vi "Image Aqq Module Test.vi"() -> ()   [LabVIEW 2015]
uses:
  <vilib>/vision/Image Controls.llb/IMAQ Image.ctl
panel:
  out "Image":T1(plugin-control)
  in  "Stop":bool
  in  "Pause":bool
  in  "Start":bool
  # "Image Stream"
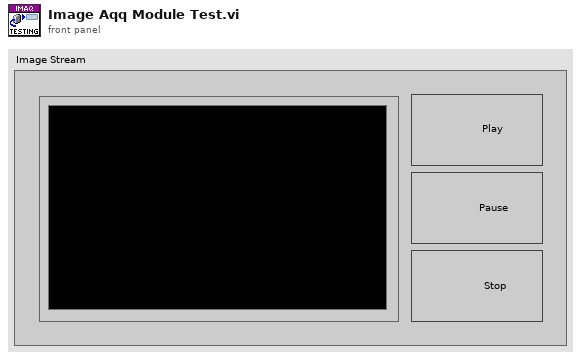
[diagram p1: front panel]
types:
  T1 = typedef "IMAQ Image.ctl" = refnum<image>
  T2 = typedef "IMAQdx.ctl" = refnum<k21>
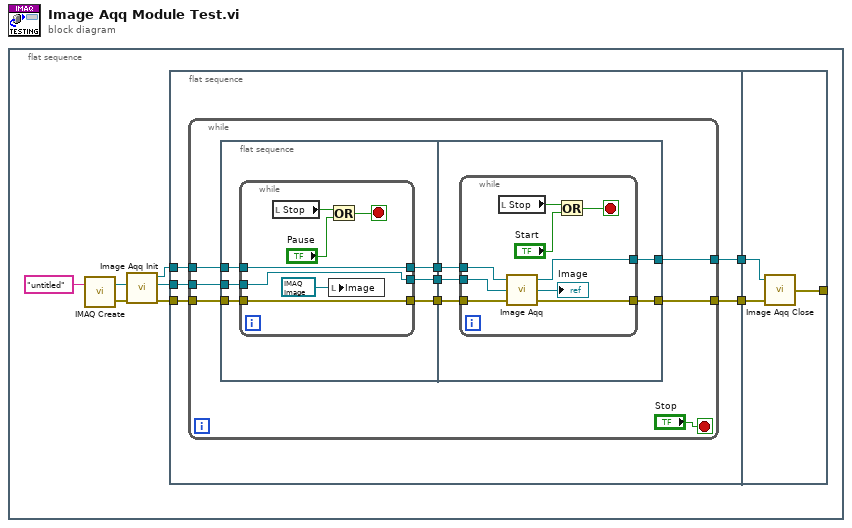
[diagram p0: block diagram]
diagram:
  n1 = flat-sequence {
    frame #0 {
      n2 = call "IMAQ Create"("Image Name"="untitled") -> ("New Image"=w5:T1, "error out"=w4:errorcluster)  [unwired: 4 in]
      n3 = call "Image Aqq Init.vi"("Error In"=w4, "Img In"=w5) -> ("Error Out"=w7:errorcluster, "Img Out"=w6:T1, "Cam Out"=w8:T2)  [unwired: 3 in]
      n4 = flat-sequence {
        tunnel: w8 -> [w13]
        tunnel: w7 -> [w12]
        tunnel: w6 -> [w11]
        tunnel: [w10] -> w2
        tunnel: [w9] -> w1
        tunnel: [w52] -> _
        tunnel: w2 -> [w51]
        tunnel: w1 -> [w50]
        frame #0 {
          n5 = while {
            tunnel: w13 -> [w18]
            tunnel: w12 -> [w15]
            tunnel: w11 -> [w19]
            tunnel: [w22] -> w10
            tunnel: [w21] -> w9
            stop <- "Stop" stop-if-true
            n6 = flat-sequence {
              tunnel: [w28] -> w20
              tunnel: w19 -> [w27]
              tunnel: w18 -> [w26]
              tunnel: [w25] -> w17
              tunnel: [w24] -> w16
              tunnel: w15 -> [w23]
              tunnel: [w40] -> w22
              tunnel: [w39] -> w21
              tunnel: w20 -> [w38]
              tunnel: w17 -> [w37]
              tunnel: w16 -> [w36]
              frame #0 {
                n7 = while {
                  tunnel: [w34] -> w28
                  tunnel: w27 -> [w34]
                  tunnel: w26 -> [w33]
                  tunnel: [w33] -> w25
                  tunnel: [w32] -> w24
                  tunnel: w23 -> [w32]
                  stop <- w35 stop-if-true
                  n8 = local read "Stop"() -> (w30:bool)
                  n9 = Or(x=w30, y="Pause") -> (x .or. y?=w35:bool)
                  n10 = local write "Image"(T1 refnum) -> ()
                }
              }
              frame #1 {
                n11 = while {
                  tunnel: [w48] -> w40
                  tunnel: [w47] -> w39
                  tunnel: w38 -> [w46]
                  tunnel: w37 -> [w45]
                  tunnel: w36 -> [w44]
                  stop <- w49 stop-if-true
                  n12 = local read "Stop"() -> (w42:bool)
                  n13 = call "Image Aqq.vi"("Error In"=w44, "Img In"=w46, "Session In"=w45) -> ("Error Out"=w48:errorcluster, "Image"=→"Image":T1, "Cam Out"=w47:T2)
                  n14 = Or(x=w42, y="Start") -> (x .or. y?=w49:bool)
                }
              }
            }
          }
        }
        frame #1 {
          n15 = call "Image Aqq Close.vi"("Error In"=w51, "Session In"=w50) -> ("Error Out"=w52:errorcluster)  [unwired: 1 in]
        }
      }
    }
  }
